vi "sensor value to pp string.vi"(8 "error in (no error)":errorcluster, 9 "strbuffer_len":u64, 10 "pp_string_out":string, 11 "h":u64) -> (0 "error out":errorcluster, 2 "pp_string_out out":string, 3 "function return":u32(ring))   [LabVIEW 2023, in "uhd.lvlib"]
doc: "UHD_API uhd_error uhd_sensor_value_to_pp_string(\n uhd_sensor_value_handle h, char* pp_string_out, size_t strbuffer_len);"
uses:
  <userlib>/uhd/uhd.lvlib
  <userlib>/uhd/uhd.dll
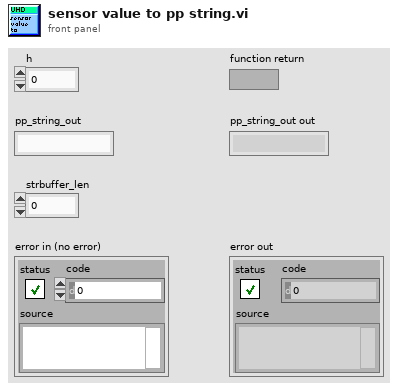
[diagram p1: front panel]
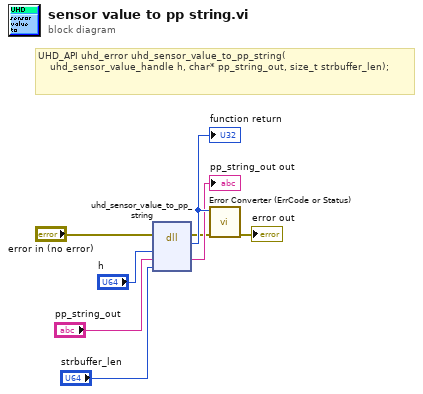
[diagram p0: block diagram]
diagram:
  # "UHD_API uhd_error uhd_sensor_value_to_pp_string(\n    uhd_sensor_value_handle h, char* pp_string_out, size_t strbuffer_len);"
  n1 = dll-call lib="C:/Program Files/National Instruments/LabVIEW 2023/user.lib/uhd/uhd.*" fn="uhd_sensor_value_to_pp_string"(error in="error in (no error)", "h"="h", "pp_string_out"="pp_string_out", "strbuffer_len"="strbuffer_len") -> (error out=w2:errorcluster, w8:u32, "pp_string_out"=→"pp_string_out out":string)  [unwired: 4 in, 1 out]
  "function return" <- w8
  n2 = call <userlib>:"Error Converter (ErrCode or Status).vi"("error in (no error)"=w2, "error code"=w8) -> ("error out"=→"error out":errorcluster)  [unwired: 9 in]
